vi "Init.vi"(8 "error in (no error)":errorcluster, 11 "Debug":bool) -> (0 "error out":errorcluster, 3 "NoControllerException out":refnum<class "NoControllerException.lvclass">)   [LabVIEW 2020, in "HTTP Server.lvlib" / "NoControllerException.lvclass"]
uses:
  NoControllerException.lvclass
  NoControllerException.lvclass/NoControllerException.ctl
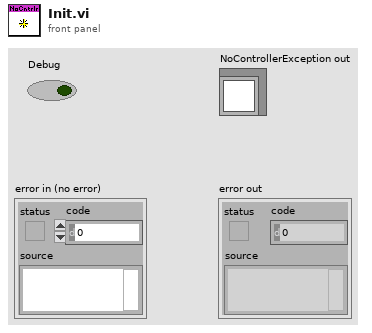
[diagram p1: front panel]
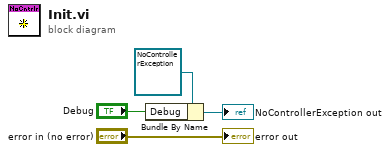
[diagram p0: block diagram]
diagram:
  n1 = Bundle By Name(cluster=refnum<class "NoControllerException.lvclass"> refnum ("NoControllerException out"), "Debug"="Debug") -> (→"NoControllerException out":refnum<class "NoControllerException.lvclass">)
  "error out" <- "error in (no error)"
